vi "run.vi"(8 "error in (no error)":errorcluster, 11 "DL090211FrameImageAssembler in":refnum<class "ImageAssemblerDL090211Scaffold.lvclass">) -> (0 "error out":errorcluster, 3 "DL090211FrameImageAssembler out":refnum<class "ImageAssemblerDL090211Scaffold.lvclass">)   [LabVIEW 2010, in "ImageAssemblerDL090211Scaffold.lvclass"]
uses:
  ImageAssemblerDL090211Scaffold.lvclass
  action_enum.ctl
  GenericImageAssembler/GenericImageAssembler/GenericImageAssembler.lvclass
  common/classes/ErrorController/ErrorController/class_data.vi
  common/classes/ErrorController/ErrorController/ErrorController.lvclass
panel:
  out "last trigger":T1
  out "statechart error":errorcluster
  out "statechart loop counter":i32
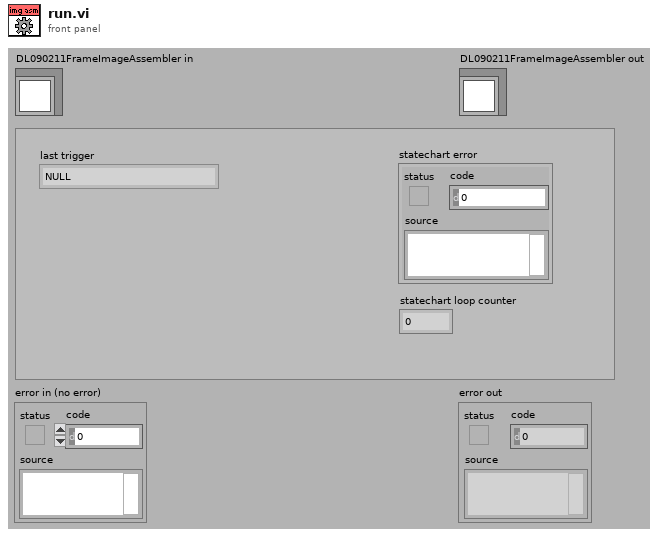
[diagram p1: front panel]
types:
  T1 = typedef "ImageAssemblerDL090211Scaffold.lvclass/action_enum.ctl" = enum16{"NULL", "initialise", "terminate", "start", "stop", "insert", "send", "attach observer", "register as observer", "detach observer"}
  T2 = typedef "top-level_component_type_enum.ctl" = enum16{"undefined", "ImagingMode", "ScanHead", "DAQ", "ImageAssembler", "Display", "DataCollection", "Analyser", "Stimulator", "ExperimentController", "Instrument", "Stage"}
  T3 = typedef "main_trigger_enum.ctl" = enum16{"NULL", "initialise", "terminate", "start", "stop", "change objective", "change experimentController", "change imagingMode", "save notebook", "started saving", "finished saving", "expCtr ready", "expCtr missing", "imgMd ready", "imgMd missing", "scanHd ready", "scanHd missing", "DAQ ready", "DAQ missing", "imgAsm ready", "imgAsm missing", "dataColl ready", "dataColl missing", "display ready", "display missing", "analysr ready", "analysr missing", "instrmnt ready", "instrmnt missing", "stimltr ready", "stimltr missing", "stage ready", "stage missing"}
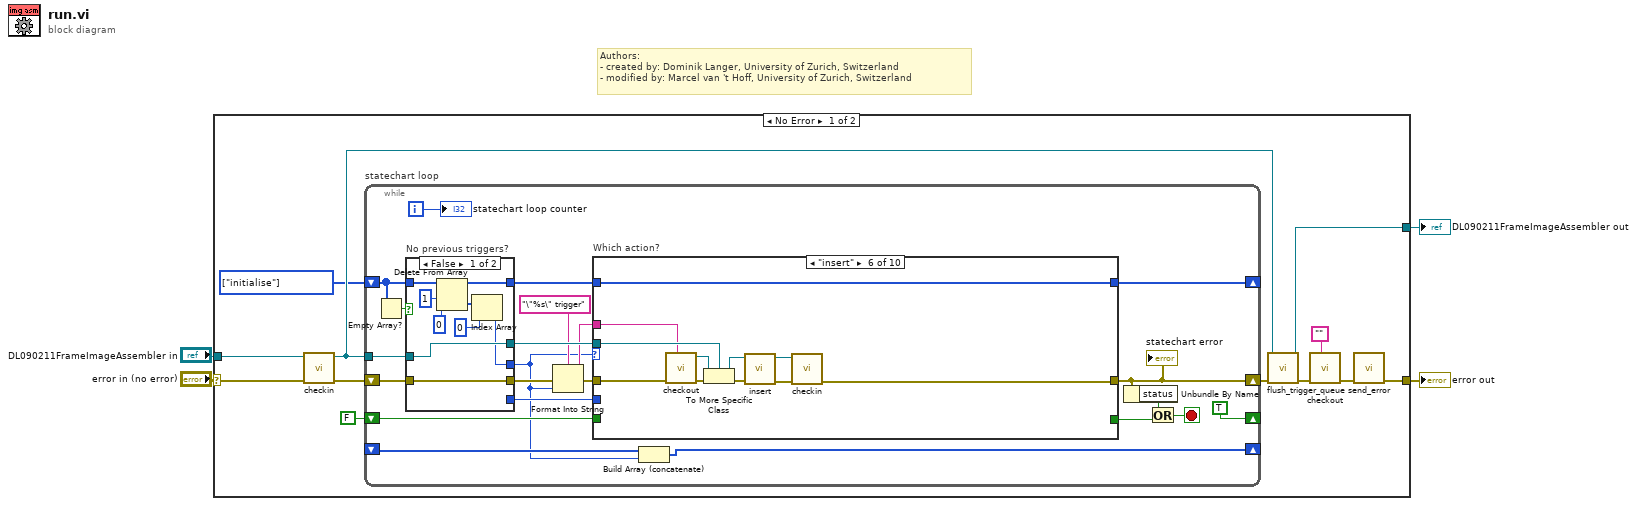
[diagram p0: block diagram]
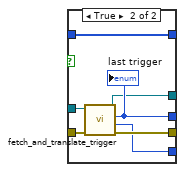
[diagram p2: hidden frame]
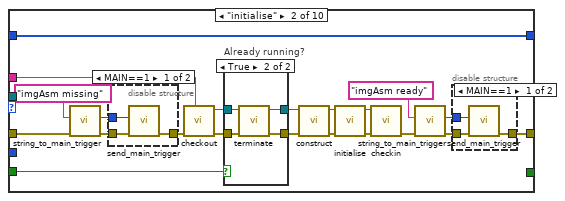
[diagram p4: hidden frame]
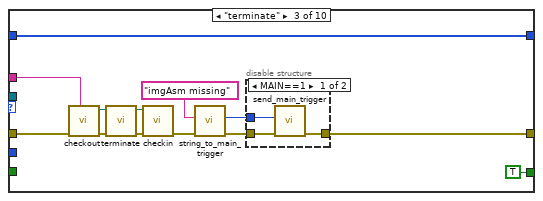
[diagram p8: hidden frame]
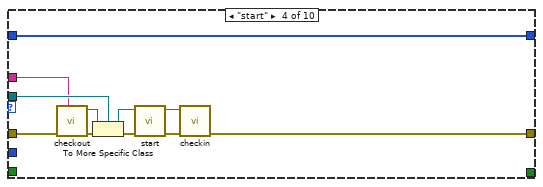
[diagram p10: hidden frame]
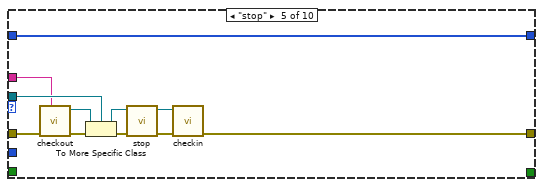
[diagram p11: hidden frame]
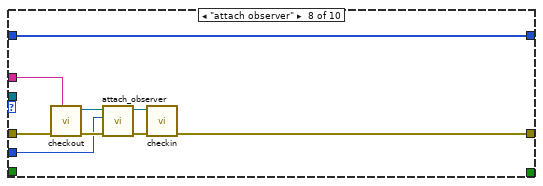
[diagram p13: hidden frame]
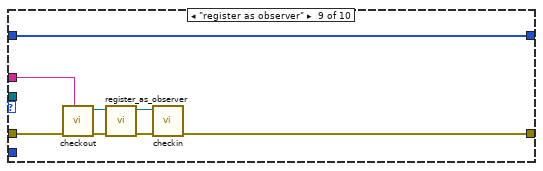
[diagram p14: hidden frame]
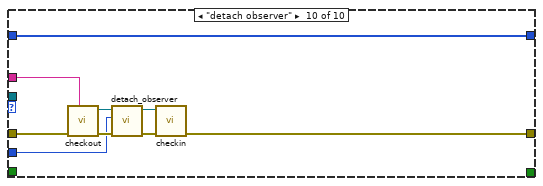
[diagram p15: hidden frame]
diagram:
  # "Authors: \n- created by: Dominik Langer, University of Zurich, Switzerland\n- modified by: Marcel van 't Hoff, University of Zurich, Switzerland"
  n1 = case shown="No Error" "error in (no error)" {
    selector: "error in (no error)" -> [w14 w171]
    tunnel: [w8 w171] -> w3
    tunnel: [w11 w170] -> w1
    tunnel: "DL090211FrameImageAssembler in" -> [w13 w170]
    frame No Error {
      w5 = T1[] [enum."initialise"] items=["NULL", "initialise", "terminate", "start", "stop", "insert", "send", "attach observer", "register as observer", "detach observer"]
      n2 = call-dynamic "checkin.vi"("error in (no error)"=w14, "GenericImageAssembler in"=w13) -> ("error out"=w6:errorcluster, "GenericImageAssembler out"=w7:refnum<class "ImageAssemblerDL090211Scaffold.lvclass">)  [unwired: 8 in]
      n3 = while "statechart loop" {
        shift-right: [w32] -> w12
        shift-left: w6 -> [w37]
        shift-right: [TRUE] -> _
        shift-left: FALSE -> [w28]
        tunnel: w7 -> [w36]
        shift-right: [w27] -> _
        shift-left: w5 -> [w25]
        shift-right: [w17] -> _
        shift-left: _ -> [w19]
        i -> [w38]
        stop <- w35 stop-if-true
        n4 = Empty Array?(array=w25) -> (empty?=w24:bool)
        n5 = case "No previous triggers?" shown="False" w24 {
          tunnel: w37 -> [w46 w54]
          tunnel: w36 -> [w47 w53]
          tunnel: [w40 w52] -> w18
          tunnel: [w46 w51] -> w22
          tunnel: [_ w50] -> w34
          tunnel: [w47 w49] -> w33
          tunnel: w25 -> [w45 w48]
          tunnel: [w44 w48] -> w26
          frame False {
            n6 = Delete From Array(array=w45, length=1, index=0) -> (deleted portion=w42:T1[], array with subset deleted=w44:T1[])
            n7 = Index Array(array=w42, index=0) -> (element=w40:T1)
          }
          frame True {
            n8 = call-dynamic "fetch_and_translate_trigger.vi"("error in (no error)"=w54, "ImageAssemblerDL090211Scaffold in"=w53) -> ("error out"=w51:errorcluster, "sender TLC type"=w50:T2, "internal trigger"=w52:T1, "ImageAssemblerDL090211Scaffold out"=w49:refnum<class "ImageAssemblerDL090211Scaffold.lvclass">)  [unwired: 6 in]
            "last trigger" <- w52
          }
        }
        n9 = Format Into String(format string="\"%s\" trigger", error in=w22, w18) -> (resulting string=w21:string, error out=w23:errorcluster)  [unwired: 1 in]
        n10 = case "Which action?" shown="\"insert\"" w18 {
          tunnel: w23 -> [w56 w60 w100 w113 w123 w135 w143 w148 w156 w165]
          tunnel: w34 -> [_ _ _ _ _ _ _ w146 _ w163]
          tunnel: [w56 w73 w99 w111 w122 w133 w143 w147 w155 w164] -> w32
          tunnel: w33 -> [_ _ _ w112 w124 w134 _ _ _ _]
          tunnel: [_ _ TRUE _ _ _ _ _ _ _] -> w31
          tunnel: w28 -> [_ w68 _ _ _ _ _ _ _ _]
          tunnel: w26 -> [w55 w67 w97 w110 w130 w132 w142 w145 w154 w162]
          tunnel: [w55 w67 w97 w110 w130 w132 w142 w145 w154 w162] -> w27
          tunnel: w21 -> [_ w66 w96 w109 w120 w131 _ w144 w153 w161]
          frame "NULL", Default {
          }
          frame "initialise" {
            n11 = call "string_to_main_trigger.vi"("error in (no error)"=w60, "trigger string"="imgAsm missing") -> ("error out"=w59:errorcluster, "main trigger"=w57:T3)  [unwired: 8 in]
            n12 = disable-structure shown="MAIN==1" {
              disable-tunnel: w59 -> [w80 w81]
              disable-tunnel: [w79 w81] -> w65
              disable-tunnel: w57 -> [w78 _]
              frame condition #0 (active) {
                n13 = call "send_main_trigger.vi"("error in (no error)"=w80, "trigger"=w78) -> ("error out"=w79:errorcluster)  [unwired: 9 in]
              }
              frame condition #1 {
              }
            }
            n14 = call "checkout.vi"("locked by?"=w66, "error in (no error)"=w65) -> ("error out"=w70:errorcluster, "GenericImageAssembler out"=w72:refnum<class "GenericImageAssembler.lvclass">)  [unwired: 8 out]
            n15 = case "Already running?" shown="True" w68 {
              tunnel: w72 -> [w83 w87]
              tunnel: [w83 w86] -> w71
              tunnel: w70 -> [w82 w85]
              tunnel: [w82 w84] -> w69
              frame False {
              }
              frame True {
                n16 = call-dynamic "terminate.vi"("error in (no error)"=w85, "GenericPlugin in"=w87) -> ("error out"=w84:errorcluster, "GenericPlugin out"=w86:refnum<class "GenericImageAssembler.lvclass">)  [unwired: 8 out]
              }
            }
            n17 = call-dynamic "construct.vi"("error in (no error)"=w69, "GenericPlugin in"=w71) -> ("error out"=w76:errorcluster, "GenericPlugin out"=w77:refnum<class "GenericImageAssembler.lvclass">)  [unwired: 2 in, 6 out]
            n18 = call-dynamic "initialise.vi"("error in (no error)"=w76, "GenericPlugin in"=w77) -> ("error out"=w75:errorcluster, "GenericPlugin out"=w74:refnum<class "GenericImageAssembler.lvclass">)  [unwired: 8 out]
            n19 = call-dynamic "checkin.vi"("error in (no error)"=w75, "GenericImageAssembler in"=w74) -> ("error out"=w64:errorcluster)  [unwired: 8 in, 1 out]
            n20 = call "string_to_main_trigger.vi"("error in (no error)"=w64, "trigger string"="imgAsm ready") -> ("error out"=w63:errorcluster, "main trigger"=w61:T3)  [unwired: 8 in]
            n21 = disable-structure shown="MAIN==1" {
              disable-tunnel: w63 -> [w90 w91]
              disable-tunnel: [w89 w91] -> w73
              disable-tunnel: w61 -> [w88 _]
              frame condition #0 (active) {
                n22 = call "send_main_trigger.vi"("error in (no error)"=w90, "trigger"=w88) -> ("error out"=w89:errorcluster)  [unwired: 9 in]
              }
              frame condition #1 {
              }
            }
          }
          frame "terminate" {
            n23 = call "checkout.vi"("locked by?"=w96, "error in (no error)"=w100) -> ("error out"=w104:errorcluster, "GenericImageAssembler out"=w103:refnum<class "GenericImageAssembler.lvclass">)  [unwired: 8 out]
            n24 = call-dynamic "terminate.vi"("error in (no error)"=w104, "GenericPlugin in"=w103) -> ("error out"=w101:errorcluster, "GenericPlugin out"=w102:refnum<class "GenericImageAssembler.lvclass">)  [unwired: 8 out]
            n25 = call-dynamic "checkin.vi"("error in (no error)"=w101, "GenericImageAssembler in"=w102) -> ("error out"=w95:errorcluster)  [unwired: 8 in, 1 out]
            n26 = call "string_to_main_trigger.vi"("error in (no error)"=w95, "trigger string"="imgAsm missing") -> ("error out"=w94:errorcluster, "main trigger"=w92:T3)  [unwired: 8 in]
            n27 = disable-structure shown="MAIN==1" {
              disable-tunnel: [w107 w108] -> w99
              disable-tunnel: w94 -> [w106 w108]
              disable-tunnel: w92 -> [w105 _]
              frame condition #0 (active) {
                n28 = call "send_main_trigger.vi"("error in (no error)"=w106, "trigger"=w105) -> ("error out"=w107:errorcluster)  [unwired: 9 in]
              }
              frame condition #1 {
              }
            }
          }
          frame "start" {
            n29 = call "checkout.vi"("locked by?"=w109, "error in (no error)"=w113) -> ("error out"=w119:errorcluster, "GenericImageAssembler out"=w118:refnum<class "GenericImageAssembler.lvclass">)  [unwired: 8 out]
            n30 = To More Specific Class(target class=w112, reference=w118, error in=w119) -> (specific class reference=w115:refnum<class "ImageAssemblerDL090211Scaffold.lvclass">, error out=w117:errorcluster)
            n31 = call-dynamic "start.vi"("error in (no error)"=w117, "DL090211ImageAssemblerScaffold in"=w115) -> ("error out"=w116:errorcluster, "DL090211ImageAssemblerScaffold out"=w114:refnum<class "ImageAssemblerDL090211Scaffold.lvclass">)  [unwired: 8 out]
            n32 = call-dynamic "checkin.vi"("error in (no error)"=w116, "GenericImageAssembler in"=w114) -> ("error out"=w111:errorcluster)  [unwired: 8 in, 1 out]
          }
          frame "stop" {
            n33 = call "checkout.vi"("locked by?"=w120, "error in (no error)"=w123) -> ("error out"=w129:errorcluster, "GenericImageAssembler out"=w125:refnum<class "GenericImageAssembler.lvclass">)  [unwired: 8 out]
            n34 = To More Specific Class(target class=w124, reference=w125, error in=w129) -> (specific class reference=w126:refnum<class "ImageAssemblerDL090211Scaffold.lvclass">, error out=w128:errorcluster)
            n35 = call-dynamic "stop.vi"("error in (no error)"=w128, "GenericToplevelComponent in"=w126) -> ("error out"=w127:errorcluster, "GenericToplevelComponent out"=w121:refnum<class "ImageAssemblerDL090211Scaffold.lvclass">)  [unwired: 8 in]
            n36 = call-dynamic "checkin.vi"("error in (no error)"=w127, "GenericImageAssembler in"=w121) -> ("error out"=w122:errorcluster)  [unwired: 8 in, 1 out]
          }
          frame "insert" {
            n37 = call "checkout.vi"("locked by?"=w131, "error in (no error)"=w135) -> ("error out"=w141:errorcluster, "GenericImageAssembler out"=w140:refnum<class "GenericImageAssembler.lvclass">)  [unwired: 8 out]
            n38 = To More Specific Class(target class=w134, reference=w140, error in=w141) -> (specific class reference=w138:refnum<class "ImageAssemblerDL090211Scaffold.lvclass">, error out=w139:errorcluster)
            n39 = call-dynamic "insert.vi"("error in (no error)"=w139, "ImageAssemblerDL090211Scaffold in"=w138) -> ("error out"=w137:errorcluster, "ImageAssemblerDL090211Scaffold out"=w136:refnum<class "ImageAssemblerDL090211Scaffold.lvclass">)  [unwired: 8 out]
            n40 = call-dynamic "checkin.vi"("error in (no error)"=w137, "GenericImageAssembler in"=w136) -> ("error out"=w133:errorcluster)  [unwired: 8 in, 1 out]
          }
          frame "send" {
          }
          frame "attach observer" {
            n41 = call "checkout.vi"("locked by?"=w144, "error in (no error)"=w148) -> ("error out"=w152:errorcluster, "GenericImageAssembler out"=w151:refnum<class "GenericImageAssembler.lvclass">)  [unwired: 8 in]
            n42 = call-dynamic "attach_observer.vi"("error in (no error)"=w152, "top-level component type"=w146, "GenericToplevelComponent in"=w151) -> ("error out"=w149:errorcluster, "GenericToplevelComponent out"=w150:refnum<class "GenericImageAssembler.lvclass">)  [unwired: 7 in]
            n43 = call-dynamic "checkin.vi"("error in (no error)"=w149, "GenericImageAssembler in"=w150) -> ("error out"=w147:errorcluster)  [unwired: 8 in, 1 out]
          }
          frame "register as observer" {
            n44 = call "checkout.vi"("locked by?"=w153, "error in (no error)"=w156) -> ("error out"=w158:errorcluster, "GenericImageAssembler out"=w157:refnum<class "GenericImageAssembler.lvclass">)  [unwired: 8 in]
            n45 = call-dynamic "register_as_observer.vi"("error in (no error)"=w158, "GenericToplevelComponent in"=w157) -> ("error out"=w160:errorcluster, "GenericToplevelComponent out"=w159:refnum<class "GenericImageAssembler.lvclass">)  [unwired: 8 in]
            n46 = call-dynamic "checkin.vi"("error in (no error)"=w160, "GenericImageAssembler in"=w159) -> ("error out"=w155:errorcluster)  [unwired: 8 in, 1 out]
          }
          frame "detach observer" {
            n47 = call "checkout.vi"("locked by?"=w161, "error in (no error)"=w165) -> ("error out"=w169:errorcluster, "GenericImageAssembler out"=w168:refnum<class "GenericImageAssembler.lvclass">)  [unwired: 8 in]
            n48 = call-dynamic "detach_observer.vi"("error in (no error)"=w169, "top-level component type"=w163, "GenericToplevelComponent in"=w168) -> ("error out"=w166:errorcluster, "GenericToplevelComponent out"=w167:refnum<class "GenericImageAssembler.lvclass">)  [unwired: 7 in]
            n49 = call-dynamic "checkin.vi"("error in (no error)"=w166, "GenericImageAssembler in"=w167) -> ("error out"=w164:errorcluster)  [unwired: 8 in, 1 out]
          }
        }
        "statechart error" <- w32
        n50 = Build Array (concatenate)(w19, w18) -> (w17:T1[])
        n51 = Unbundle By Name(w32) -> ("status"=w30:bool)
        n52 = Or(x=w30, y=w31) -> (x .or. y?=w35:bool)
        "statechart loop counter" <- w38
      }
      n53 = call-dynamic "flush_trigger_queue.vi"("error in (no error)"=w12, "GenericToplevelComponent in"=w7) -> ("error out"=w10:errorcluster, "GenericToplevelComponent out"=w11:refnum<class "ImageAssemblerDL090211Scaffold.lvclass">)  [unwired: 8 in]
      n54 = call "checkout.vi"("locked by?"="", "error in (no error)"=w10) -> ("error out"=w9:errorcluster)  [unwired: 9 out]
      n55 = call "send_error.vi"("error in (no error)"=w9) -> ("error out"=w8:errorcluster)  [unwired: 10 in]
    }
    frame Error {
    }
  }
  "error out" <- w3
  "DL090211FrameImageAssembler out" <- w1
